vi "Peak.vi"(11 "TypedCircularBuffer in":refnum<class "TypedCircularBuffer.lvclass">) -> (2 "element":T1, 3 "TypedCircularBuffer out":refnum<class "TypedCircularBuffer.lvclass">)   [LabVIEW 2024, in "TypedCircularBuffer.lvclass"]
uses:
  TypedCircularBuffer.lvclass
  Type.ctl
  TypedCircularBuffer.lvclass/TypedCircularBuffer.ctl
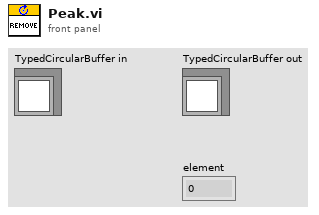
[diagram p1: front panel]
types:
  T1 = typedef "TypedCircularBuffer.lvclass/Type.ctl" = i32
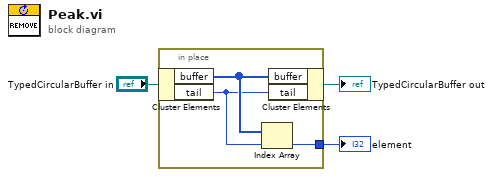
[diagram p0: block diagram]
diagram:
  n1 = in-place {
    in-place-border: [w5] -> w1
    n2 = in-place-cluster #1("TypedCircularBuffer in") -> ("buffer"=w6:T1[], "tail"=w4:u32)
    n3 = Index Array(array=w6, index=w4) -> (element=w5:T1)
    n4 = in-place-cluster #1("buffer"=w6, "tail"=w4) -> (→"TypedCircularBuffer out":refnum<class "TypedCircularBuffer.lvclass">)
  }
  "element" <- w1
